vi "SnapshotHasID.vi"(8 "id":string, 11 "Snapshot":T1={"globalThreshold"=enum."INFO", "appenders"=[]}) -> (3 "found":bool)   [LabVIEW 2026, in "Lumberjack.lvlib" / "Logger.lvclass"]
doc: "Returns whether an appender with the given id is present in a published Snapshot. Scans the Snapshot's appenders array for an exact id match and short-circuits on the first hit. Used by WaitForSnapshot to evaluate the IDPresent/IDAbsent conditions, and available to tests asserting registry membership. Pure: no state, no side effects."
uses:
  Logger.lvclass
  TypeDefs/Snapshot.ctl
  TypeDefs/Severity.ctl
  <vilib>/ActorFramework/Message Enqueuer/Message Enqueuer.lvclass
  Lumberjack.lvlib
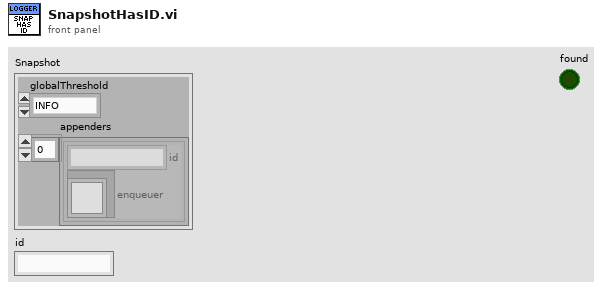
[diagram p1: front panel]
types:
  T1 = typedef "Lumberjack.lvlib/Snapshot.ctl" = cluster{"globalThreshold":T2, "appenders":cluster{"id":string, "enqueuer":refnum<class "Message Enqueuer.lvclass">}[]}
  T2 = typedef "Lumberjack.lvlib/Severity.ctl" = enum16{"OFF", "FATAL", "ERROR", "WARN", "INFO", "DEBUG", "TRACE", "ALL"}
  T3 = cluster{"id":string, "enqueuer":refnum<class "Message Enqueuer.lvclass">}[]
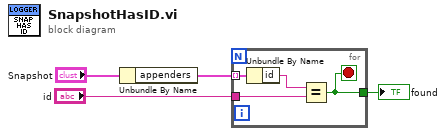
[diagram p0: block diagram]
diagram:
  n1 = Unbundle By Name("Snapshot") -> ("appenders"=w3:T3)
  n2 = for {
    tunnel: w3 -> [w8] mode=indexing
    tunnel: "id" -> [w6]
    tunnel: [w5] -> w1
    stop <- w5 stop-if-true
    n3 = Unbundle By Name(w8) -> ("id"=w7:string)
    n4 = Equal?(x=w7, y=w6) -> (x = y?=w5:bool)
  }
  "found" <- w1
